vi "RawUnitsToRPM-2048-CPR.vi"(2 "Gear Ratio":dbl=1.0, 3 "Raw Units":i32) -> (0 "RPM":dbl)   [LabVIEW 2020, in "TitanLib.lvlib"]
uses:
  TitanLib.lvlib
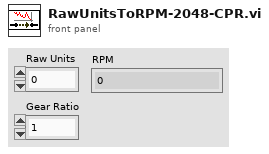
[diagram p1: front panel]
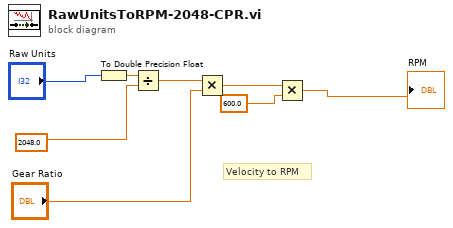
[diagram p0: block diagram]
diagram:
  # "Velocity to RPM"
  n1 = To Double Precision Float(number="Raw Units") -> (double precision float=w5:dbl)
  n2 = Divide(x=w5, y=2048.0) -> (x/y=w3:dbl)
  n3 = Multiply(x=w3, y="Gear Ratio") -> (x*y=w2:dbl)
  n4 = Multiply(x=w2, y=600.0) -> (x*y=→"RPM":dbl)
